vi "json Parse Path - string path.vi"(8 "error in (no error)":errorcluster, 9 "default":path, 10 "path":string, 11 "JSON Document in":refnum<class "JSON Document.lvclass">) -> (0 "error out":errorcluster, 2 "value":path, 3 "JSON Document out":refnum<class "JSON Document.lvclass">)   [LabVIEW 2015, in "JSON Document.lvclass"]
uses:
  JSON Document.lvclass
  JSON Document.lvclass/JSON Document.ctl
  rapidjson wrapper/rapidjson wrapper.lvlib
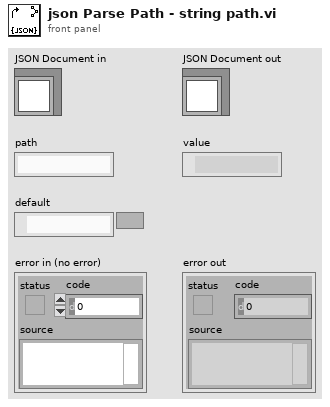
[diagram p1: front panel]
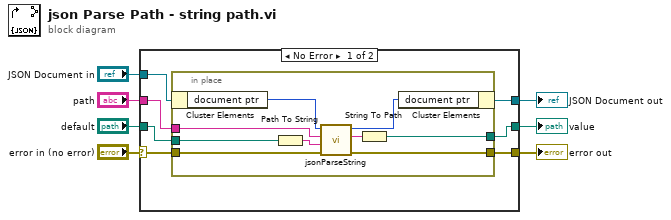
[diagram p0: block diagram]
diagram:
  n1 = case shown="No Error" "error in (no error)" {
    selector: "error in (no error)" -> [w11 w26]
    tunnel: [w10 w26] -> w6
    tunnel: [w9 w25] -> w4
    tunnel: "JSON Document in" -> [w14 w25]
    tunnel: "default" -> [w13 w24]
    tunnel: "path" -> [w12 _]
    tunnel: [w8 w24] -> w1
    frame No Error {
      n2 = in-place {
        in-place-border: w13 -> [w18]
        in-place-border: w12 -> [w21]
        in-place-border: w11 -> [w20]
        in-place-border: [w19] -> w10
        in-place-border: [w15] -> w8
        n3 = in-place-cluster #1(w14) -> ("document ptr"=w23:i64)
        n4 = Path To String(path=w18) -> (string=w17:string)
        n5 = call "jsonParseString.vi"("error in (no error)"=w20, "default"=w17, "path"=w21, "d in"=w23) -> ("error out"=w19:errorcluster, "value"=w16:string, "d out"=w22:i64)  [unwired: 5 in]
        n6 = String To Path(string=w16) -> (path=w15:path)
        n7 = in-place-cluster #1("document ptr"=w22) -> (w9:refnum<class "JSON Document.lvclass">)
      }
    }
    frame Error {
    }
  }
  "error out" <- w6
  "JSON Document out" <- w4
  "value" <- w1
